vi "FTW-Package-Request-WriteResponse.vi"(8 "error in":errorcluster, 9 "Response Body":string, 11 "FTW Incoming Request":refnum<class "FTW-Package-IncomingRequest.lvclass">) -> (0 "error out":errorcluster, 3 "FTW Incoming Request out":refnum<class "FTW-Package-IncomingRequest.lvclass">)   [LabVIEW 2013, in "FTW-Package-IncomingRequest.lvclass"]
uses:
  FTW-Package-IncomingRequest.lvclass
  FTW-Package-IncomingRequest.lvclass/FTW-Package-IncomingRequest.ctl
panel:
  # "Inputs"
  # "Outputs"
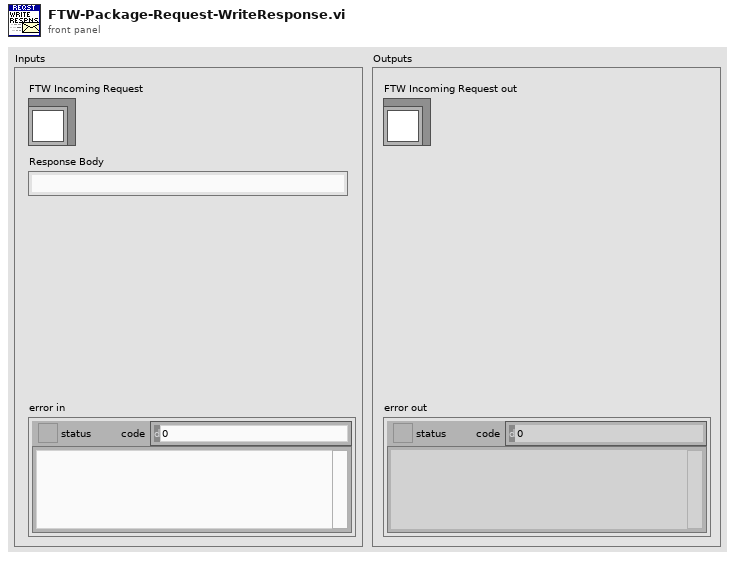
[diagram p1: front panel]
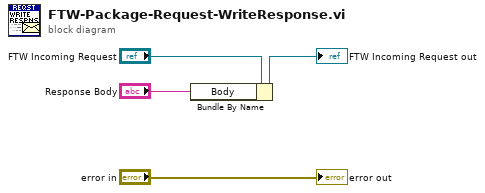
[diagram p0: block diagram]
diagram:
  n1 = Bundle By Name(cluster="FTW Incoming Request", "Body"="Response Body") -> (→"FTW Incoming Request out":refnum<class "FTW-Package-IncomingRequest.lvclass">)
  "error out" <- "error in"
